vi "Frameremap_flt.vi"(8 "FH":dbl, 9 "FW":dbl, 10 "FO Z":dbl, 11 "FO X":dbl) -> (0 "FH":dbl, 1 "FW":dbl, 2 "Z Origin":dbl, 3 "X Origin":dbl)   [LabVIEW 2017]
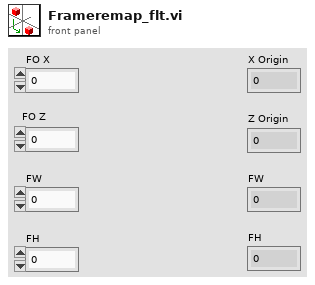
[diagram p1: front panel]
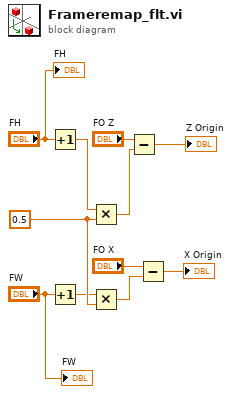
[diagram p0: block diagram]
diagram:
  w11 = 0.5 ("y")
  n1 = Increment(x="FH") -> (x+1=w1:dbl)
  n2 = Increment(x="FW") -> (x+1=w2:dbl)
  n3 = Multiply(x=w1, y=w11) -> (x*y=w7:dbl)
  n4 = Multiply(x=w2, y=w11) -> (x*y=w10:dbl)
  n5 = Subtract(x="FO Z", y=w7) -> (x-y=→"Z Origin":dbl)
  n6 = Subtract(x="FO X", y=w10) -> (x-y=→"X Origin":dbl)
  "FW" <- "FW"
  "FH" <- "FH"
